vi "Image-GFV.vi"(8 "error in (no error)":errorcluster, 10 "Input Image":T1, 11 "Image GFV Enum":T2=enum."Write") -> (0 "error out":errorcluster, 3 "Output Image":T1)   [LabVIEW 2013]
doc: "Use this template to build a VI to use as a subVI."
uses:
  ImageEnum4GFV.ctl
  <vilib>/vision/Image Controls.llb/IMAQ Image.ctl
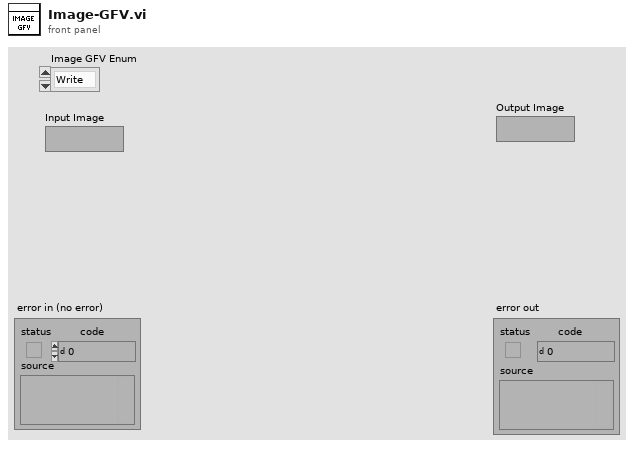
[diagram p1: front panel]
types:
  T1 = typedef "IMAQ Image.ctl" = refnum<image>
  T2 = typedef "ImageEnum4GFV.ctl" = enum16{"Delete", "Write", "Read", "Init"}
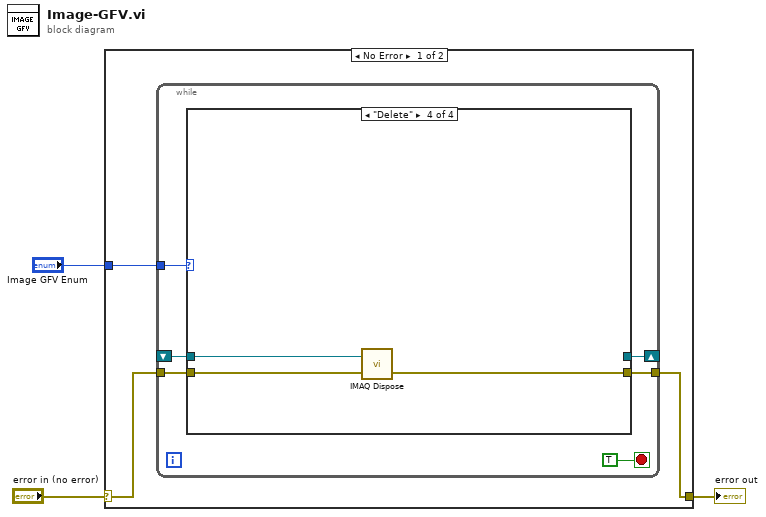
[diagram p0: block diagram]
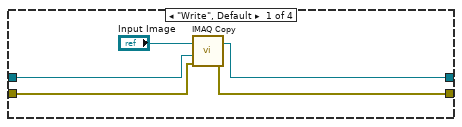
[diagram p2: hidden frame]
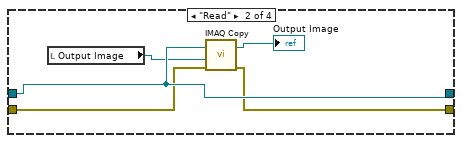
[diagram p3: hidden frame]
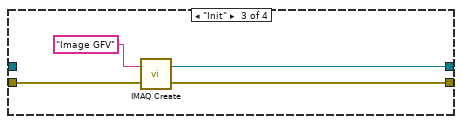
[diagram p4: hidden frame]
diagram:
  n1 = case shown="No Error" "error in (no error)" {
    selector: "error in (no error)" -> [w5 w30]
    tunnel: [w4 w30] -> w2
    tunnel: "Image GFV Enum" -> [w6 _]
    frame No Error {
      n2 = while {
        tunnel: w6 -> [w11]
        tunnel: w5 -> [w10]
        tunnel: [w9] -> w4
        shift-right: [w8] -> _
        shift-left: _ -> [w7]
        stop <- TRUE stop-if-true
        n3 = case shown="\"Delete\"" w11 {
          tunnel: w10 -> [w14 w19 w25 w29]
          tunnel: [w13 w18 w24 w28] -> w9
          tunnel: [w15 w22 w23 _] -> w8
          tunnel: w7 -> [w16 w22 _ w27]
          frame "Write", Default {
            n4 = call "IMAQ Copy"("error in (no error)"=w14, "Image Dst"=w16, "Image Src"="Input Image") -> ("error out"=w13:errorcluster, "Image Dst Out"=w15:T1)  [unwired: 3 in]
          }
          frame "Read" {
            n5 = local read "Output Image"() -> (w21:T1)
            n6 = call "IMAQ Copy"("error in (no error)"=w19, "Image Dst"=w21, "Image Src"=w22) -> ("error out"=w18:errorcluster, "Image Dst Out"=→"Output Image":T1)  [unwired: 3 in]
          }
          frame "Init" {
            n7 = call "IMAQ Create"("Image Name"="Image GFV", "error in (no error)"=w25) -> ("New Image"=w23:T1, "error out"=w24:errorcluster)  [unwired: 2 in, 1 out]
          }
          frame "Delete" {
            n8 = call "IMAQ Dispose"("Image"=w27, "error in (no error)"=w29) -> ("error out"=w28:errorcluster)  [unwired: 1 in, 3 out]
          }
        }
      }
    }
    frame Error {
    }
  }
  "error out" <- w2
